vi "LogIn Infor.vi"(8 "error in (no error)":errorcluster caption="에러 입력(에러 없음)", 11 "USER IN":T1) -> (0 "error out":errorcluster caption="에러 출력", 2 "Admin?":bool, 3 "USER OUT":T1)   [LabVIEW 2019]
uses:
  cmd_logInfor.ctl
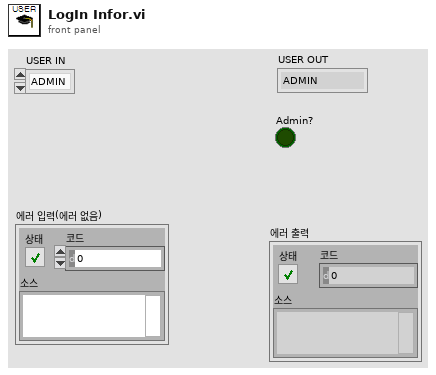
[diagram p1: front panel]
types:
  T1 = typedef "cmd_logInfor.ctl" = enum16{"ADMIN", "OPER", "DEFAULT"}
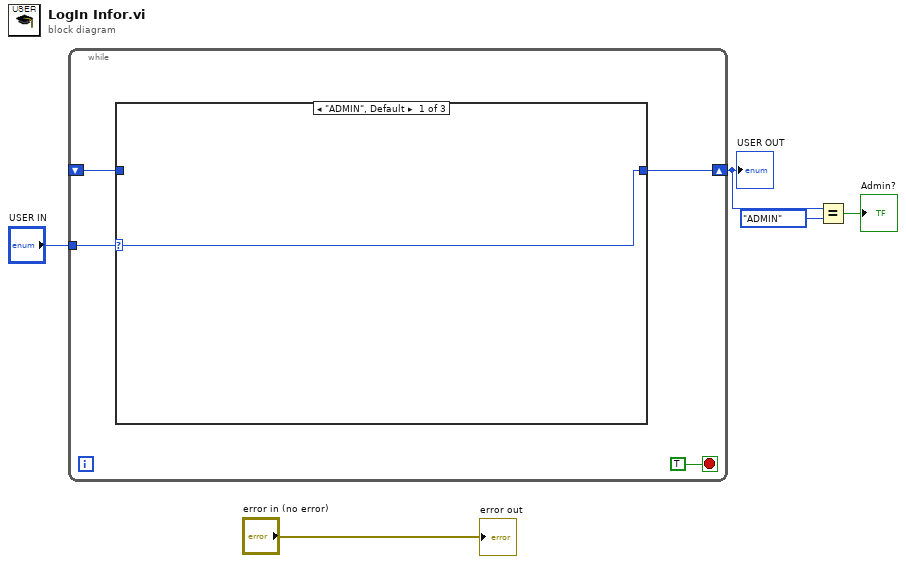
[diagram p0: block diagram]
diagram:
  n1 = while {
    tunnel: "USER IN" -> [w8]
    shift-right: [w7] -> w3
    shift-left: _ -> [w6]
    stop <- TRUE stop-if-true
    n2 = case shown="\"ADMIN\", Default" w8 {
      selector: w8 -> [w10 w11 _]
      tunnel: [w10 w11 w12] -> w7
      tunnel: w6 -> [_ _ w12]
      frame "ADMIN", Default {
      }
      frame "OPER" {
      }
      frame "DEFAULT" {
      }
    }
  }
  "USER OUT" <- w3
  n3 = Equal?(x=w3, y=cmd_logInfor."ADMIN") -> (x = y?=→"Admin?":bool)
  "error out" <- "error in (no error)"
